vi "Day 07 (Part One).vi"() -> ()   [LabVIEW 2021]
uses:
  4279ecf5-67f9-43a7-b6b3-78b14aefd003.vi
  4046d748-ad09-4f5d-82b9-a1e726cceff7.vi
  <userlib>/_OpenG.lib/array/array.llb/Sort 2D Array (I32)__ogtk.vi
  <vilib>/Comparison/Less/Less Functor/Less Functor.lvclass
panel:
  out "result":i32
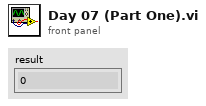
[diagram p1: front panel]
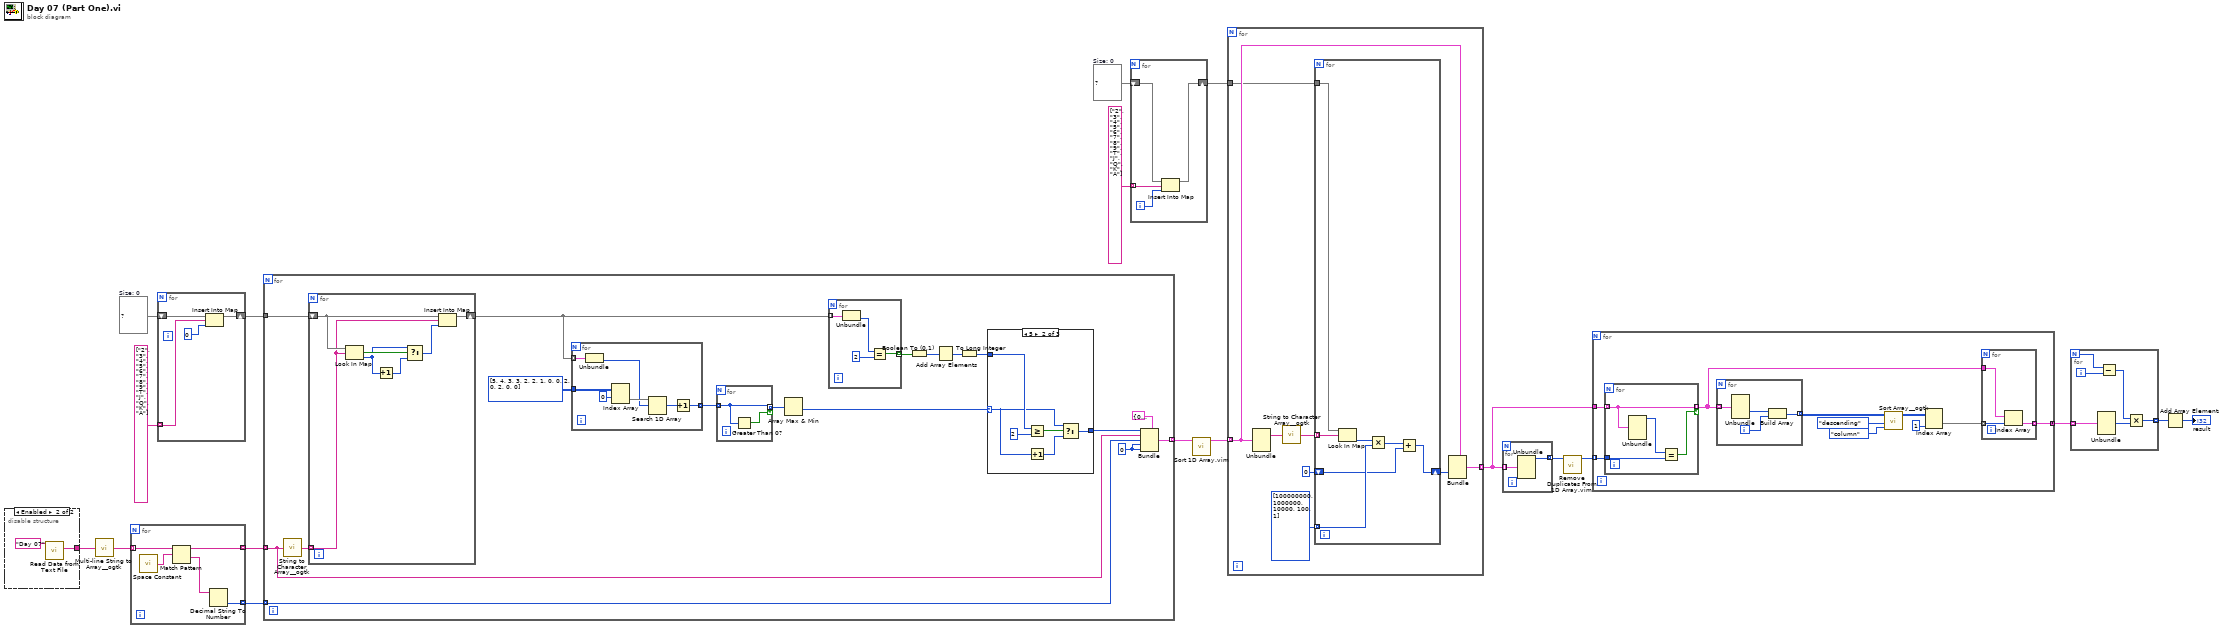
[diagram p0: block diagram]
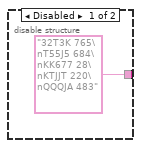
[diagram p2: hidden frame]
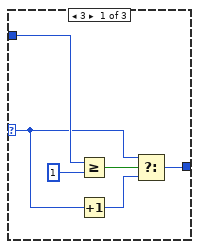
[diagram p3: hidden frame]
diagram:
  w3 = map{string, i32} {}  # Size: 0
  w15 = map{string, i32} {}  # Size: 0
  n1 = disable-structure shown="Enabled" {
    disable-tunnel: ["32T3K 765\nT55J5 684\nKK677 28\nKTJJT 220\nQQQJA 483" w21] -> w18
    frame Disabled {
    }
    frame Enabled {
      n2 = call "Read Data from Text File.vi"("Subfolder"="Day 07") -> ("data"=w21:string)  [unwired: 10 in]
    }
  }
  n3 = call <userlib>:"Multi-line String to Array__ogtk.vi"("string"=w18) -> ("lines"=w17:string[])
  n4 = for {
    tunnel: w17 -> [w26] mode=indexing
    tunnel: [w24] -> w16 mode=indexing
    tunnel: [w22] -> w13 mode=indexing
    n5 = call <vilib>:"Space Constant.vi"() -> ("String"=w25:string)
    n6 = Match Pattern(string=w26, regular expression=w25) -> (before substring=w24:string, after substring=w23:string)  [unwired: 1 in, 2 out]
    n7 = Decimal String To Number(string=w23) -> (number=w22:i32)  [unwired: 2 in, 1 out]
  }
  n8 = for {
    shift-right: [w29] -> w4
    shift-left: w15 -> [w30]
    tunnel: string[] ["2", "3", "4", "5", "6", "7", "8", "9", "T", "J", "Q", "K", "A"] -> [w27] mode=indexing
    n9 = Insert Into Map(map in=w30, key=w27, value=0) -> (map out=w29:map{string, i32})  [unwired: 2 out]
  }
  n10 = for {
    tunnel: w16 -> [w39] mode=indexing
    tunnel: w4 -> [w46]
    tunnel: [w40] -> w14 mode=indexing
    tunnel: w13 -> [w37] mode=indexing
    w31 = 0
    n11 = call <userlib>:"String to Character Array__ogtk.vi"("Input String"=w39) -> ("Character Array"=w47:string[])
    n12 = for {
      tunnel: w47 -> [w74] mode=indexing
      shift-right: [w72] -> w45
      shift-left: w46 -> [w75]
      n13 = Look In Map(map=w75, key=w74) -> (key not found?=w78:bool, value=w76:i32)  [unwired: 1 in]
      n14 = Increment(x=w76) -> (x+1=w77:i32)
      n15 = Select(t=w76, s=w78, f=w77) -> (s? t:f=w73:i32)
      n16 = Insert Into Map(map in=w75, key=w74, value=w73) -> (map out=w72:map{string, i32})  [unwired: 2 out]
    }
    n17 = for {
      tunnel: w45 -> [w71] mode=indexing
      tunnel: i32[][] [[5, 4, 3, 3, 2, 2, 1], [0, 0, 2, 0, 2, 0, 0]] -> [w70]
      tunnel: [w65] -> w44 mode=indexing
      n18 = Unbundle(w71) -> (w67:i32)  [unwired: 1 out]
      n19 = Index Array(array=w70, index (row)=0) -> (element=w68:i32[])  [unwired: 1 in]
      n20 = Search 1D Array(1D array=w68, element=w67) -> (index of element=w66:i32)  [unwired: 1 in]
      n21 = Increment(x=w66) -> (x+1=w65:i32)
    }
    n22 = for {
      tunnel: w44 -> [w80] mode=indexing
      tunnel: [w80] -> w43 mode=indexing if=w79
      n23 = Greater Than 0?(x=w80) -> (x > 0?=w79:bool)
    }
    n24 = Array Max & Min(array=w43) -> (min value=w32:i32)  [unwired: 3 out]
    n25 = for {
      tunnel: w45 -> [w64] mode=indexing
      tunnel: [w61] -> w36 mode=indexing
      n26 = Unbundle(w64) -> (w63:i32)  [unwired: 1 out]
      n27 = Equal?(x=w63, y=2) -> (x = y?=w61:bool)
    }
    n28 = Boolean To (0,1)(Boolean=w36) -> (0, 1=w35:i16[])
    n29 = Add Array Elements(numeric array=w35) -> (sum=w34:i16)
    n30 = To Long Integer(number=w34) -> (32bit integer=w33:i32)
    n31 = case shown="5" w32 {
      selector: w32 -> [w48 w54 w60]
      tunnel: w33 -> [w51 w57 _]
      tunnel: [w49 w55 w60] -> w38
      frame 3 {
        n32 = Greater Or Equal?(x=w51, y=1) -> (x >= y?=w52:bool)
        n33 = Increment(x=w48) -> (x+1=w50:i32)
        n34 = Select(t=w48, s=w52, f=w50) -> (s? t:f=w49:i32)
      }
      frame 5 {
        n35 = Greater Or Equal?(x=w57, y=2) -> (x >= y?=w58:bool)
        n36 = Increment(x=w54) -> (x+1=w56:i32)
        n37 = Select(t=w54, s=w58, f=w56) -> (s? t:f=w55:i32)
      }
      frame Default {
      }
    }
    n38 = Bundle(cluster=cluster{i32, string, i32, i32, i32} {0, "", 0, 0, 0}, w38, w39, w37, w31, w31) -> (w40:cluster{i32, string, i32, i32, i32})
  }
  n39 = for {
    shift-right: [w81] -> w1
    shift-left: w3 -> [w82]
    tunnel: string[] ["2", "3", "4", "5", "6", "7", "8", "9", "T", "J", "Q", "K", "A"] -> [w84] mode=indexing
    i -> [w83]
    n40 = Insert Into Map(map in=w82, key=w84, value=w83) -> (map out=w81:map{string, i32})  [unwired: 2 out]
  }
  n41 = call "Sort 1D Array.vim"("unsorted array"=w14) -> ("sorted array"=w12:cluster{i32, string, i32, i32, i32}[])  [unwired: 10 in]
  n42 = for {
    tunnel: w12 -> [w88] mode=indexing
    tunnel: [w86] -> w9 mode=indexing
    tunnel: w1 -> [w85]
    n43 = Unbundle(w88) -> (w92:string)  [unwired: 4 out]
    n44 = call <userlib>:"String to Character Array__ogtk.vi"("Input String"=w92) -> ("Character Array"=w91:string[])
    n45 = for {
      tunnel: w91 -> [w97] mode=indexing
      tunnel: i32[] [100000000, 1000000, 10000, 100, 1] -> [w98] mode=indexing
      shift-right: [w96] -> w87
      shift-left: 0 -> [w94]
      tunnel: w85 -> [w93]
      n46 = Look In Map(map=w93, key=w97) -> (value=w99:i32)  [unwired: 1 in, 1 out]
      n47 = Multiply(x=w99, y=w98) -> (x*y=w95:i32)
      n48 = Add(x=w95, y=w94) -> (x+y=w96:i32)
    }
    n49 = Bundle(cluster=w88, w87) -> (w86:cluster{i32, string, i32, i32, i32})  [unwired: 4 in]
  }
  n50 = for {
    tunnel: w9 -> [w101] mode=indexing
    tunnel: [w100] -> w11 mode=indexing
    n51 = Unbundle(w101) -> (w100:i32)  [unwired: 4 out]
  }
  n52 = call "Remove Duplicates From 1D Array.vim"("array"=w11) -> ("array with duplicates removed"=w10:i32[])  [unwired: 10 in]
  n53 = for {
    tunnel: w10 -> [w110] mode=indexing
    tunnel: w9 -> [w111]
    tunnel: [w102] -> w8 mode=concatenating
    n54 = for {
      tunnel: w111 -> [w113] mode=indexing
      tunnel: w110 -> [w114]
      tunnel: [w113] -> w103 mode=indexing if=w112
      n55 = Unbundle(w113) -> (w115:i32)  [unwired: 4 out]
      n56 = Equal?(x=w115, y=w114) -> (x = y?=w112:bool)
    }
    n57 = for {
      tunnel: w103 -> [w122] mode=indexing
      tunnel: [w119] -> w109 mode=indexing
      i -> [w120]
      n58 = Unbundle(w122) -> (w121:i32)  [unwired: 4 out]
      n59 = Build Array(w121, w120) -> (w119:i32[])
    }
    n60 = call-poly <userlib>:"Sort Array__ogtk.vi"("Sort By in"=enum16{"row", "column"}."column", "Order"=enum16{"ascending", "descending"}."descending", "Array in"=w109) -> ("Sorted Array out"=w106:i32[][])  [unwired: 5 in, 3 out]
    n61 = Index Array(array=w106, index (col)=1 ("disabled index (col)")) -> (element=w104:i32[])  [unwired: 1 in]
    n62 = for {
      tunnel: w104 -> [w117] mode=indexing
      tunnel: w103 -> [w118]
      tunnel: [w116] -> w102 mode=indexing
      n63 = Index Array(array=w118, index=w117) -> (element=w116:cluster{i32, string, i32, i32, i32})
    }
  }
  n64 = for {
    N -> [w128]
    tunnel: w8 -> [w124] mode=indexing
    tunnel: [w123] -> w7 mode=indexing
    i -> [w127]
    n65 = Unbundle(w124) -> (w125:i32)  [unwired: 4 out]
    n66 = Subtract(x=w128, y=w127) -> (x-y=w126:i32)
    n67 = Multiply(x=w126, y=w125) -> (x*y=w123:i32)
  }
  n68 = Add Array Elements(numeric array=w7) -> (sum=→"result":i32)
